vi "DPID.vi"(8 "error in (no error)":errorcluster, 11 "Node Ptr":T2 format="%.0x") -> (0 "error out":errorcluster)   [LabVIEW 2024, in "Diagnostics Addon System Explorer.lvlib"]
uses:
  Diagnostics Addon System Explorer.lvlib
  <vilib>/NI VeriStand/Custom Device API/Custom Device Item Ref.ctl
  Addon Shared/Types/DPID.Rate.ctl
  Types/FG.Action.ctl
  Addon Shared/SubVIs/Constants.vi
  <vilib>/NI/NI VeriStand Advanced SysDef API/SysDef API/SysDef.Property.Set.vi
  <vilib>/NI/NI VeriStand Advanced SysDef API/_SubVIs/SysDef.Property.Set.U32.vi
  <vilib>/NI VeriStand/Custom Device API/NI VeriStand - Get Item Property.vi
  <vilib>/NI VeriStand/Custom Device API/Get Item Property (U32).vi
  <vilib>/NI/NI VeriStand Advanced SysDef API/_SubVIs/SysDef.Property.Set.U32.Array.vi
  <vilib>/NI VeriStand/Custom Device API/Get Item Property (U32 Array).vi
  <vilib>/NI VeriStand/Custom Device Tools/Custom Device Utility Library/NI VeriStand - Search for Item by GUID.vi
  <vilib>/NI VeriStand/Custom Device API/Custom Device API.lvlib
  <vilib>/NI VeriStand/Custom Device Tools/Custom Device Utility Library/Custom Device Utility Library.lvlib
  Addon Shared/Diagnostics Addon Shared.lvlib
panel:
  in  "Speed":T1
  in  "Description":string
  in  "ID":u8 format="%.0x"
  out "PIDs":i32(listbox)
  in  "SHDocVw.IWebBrowser":refnum<k7>(container)
  in  "Header":cluster{"Section Name":string}={"Section Name"="DPID Settings"}
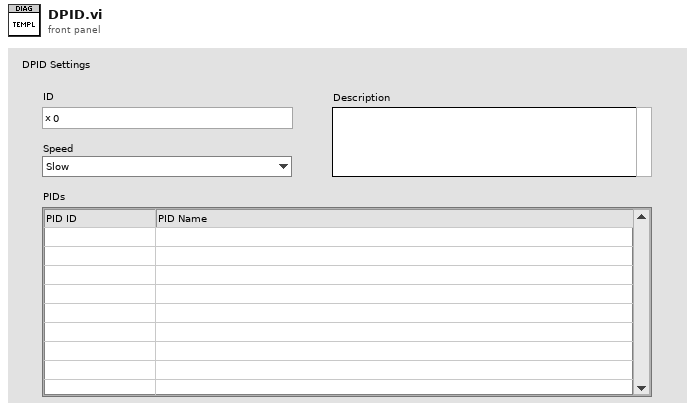
[diagram p1: front panel]
types:
  T1 = typedef "Diagnostics Addon Shared.lvlib/DPID.Rate.ctl" = enum16{"Slow", "Medium", "Fast"}
  T2 = typedef "Custom Device API.lvlib/Custom Device Item Ref.ctl" = u64
  T3 = typedef "Diagnostics Addon System Explorer.lvlib/FG.Action.ctl" = enum16{"Get", "Set"}
  T4 = typedef "Custom Device API.lvlib/Custom Device Item Info.ctl" = cluster{"Name":string, "Is Channel":bool, "GUID":string, "Is Waveform":bool}
  T5 = typedef "Diagnostics Addon Shared.lvlib/DPID.ctl" = cluster{"DPID ID":u8, "Speed":T1, "PIDs":u16[]}
  T6 = typedef "Custom Device API.lvlib/Custom Device Commands.ctl" = enum16{"Default", "Item renamed", "Shutdown", "Dynamic button pressed"}
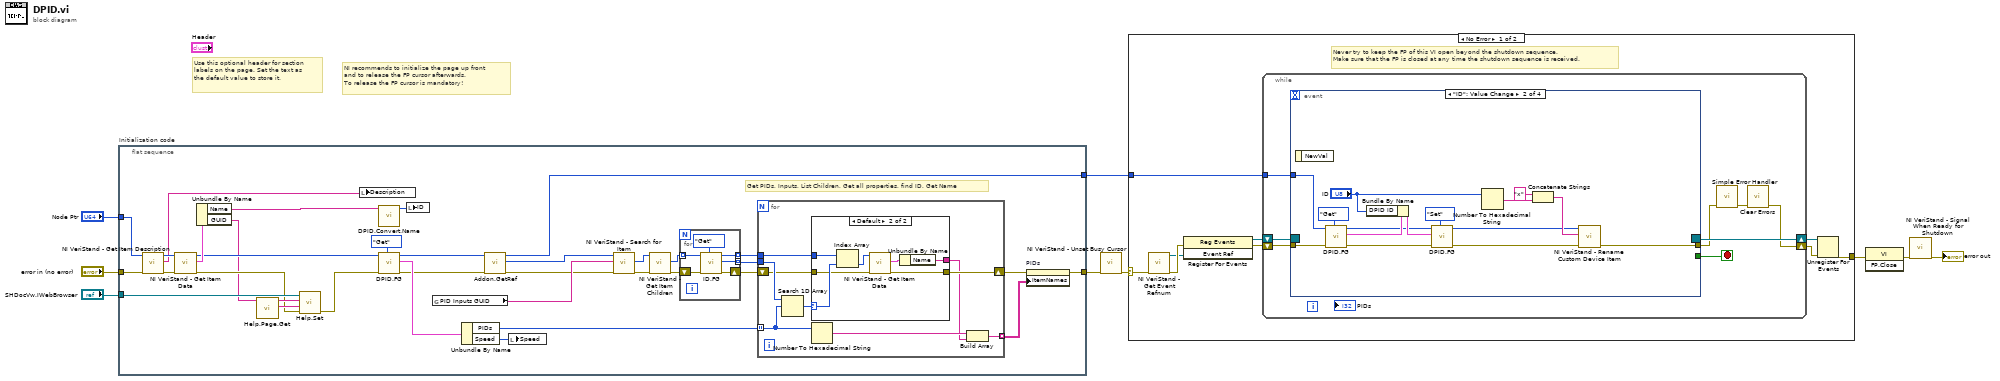
[diagram p0: block diagram]
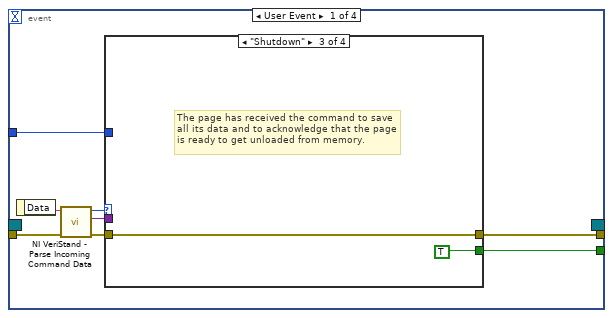
[diagram p2: hidden frame]
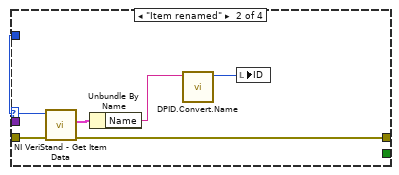
[diagram p4: hidden frame]
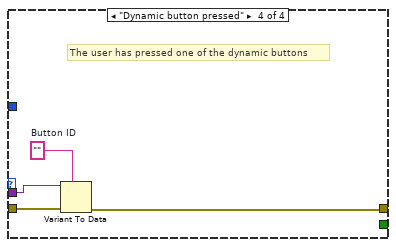
[diagram p5: hidden frame]
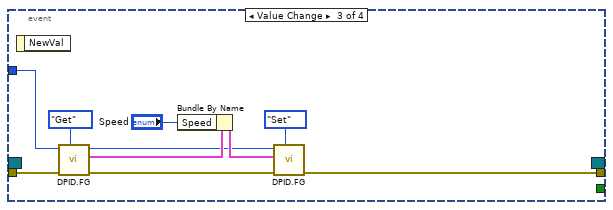
[diagram p6: hidden frame]
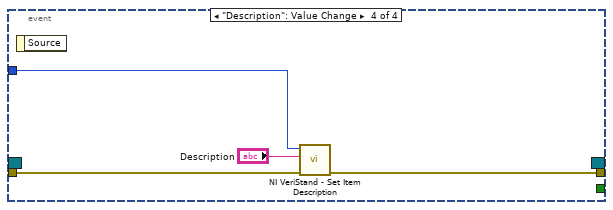
[diagram p7: hidden frame]
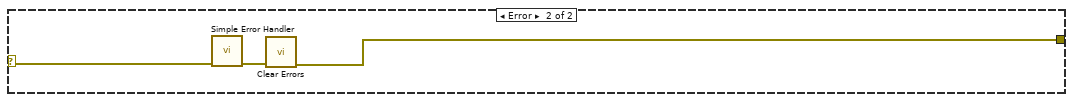
[diagram p8: hidden frame]
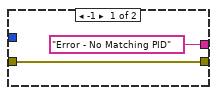
[diagram p9: hidden frame]
diagram:
  # "Use this optional header for section labels on the page. Set the text as the default value to store it."
  # "NI recommends to initialize the page up front\nand to release the FP cursor afterwards.\nTo release the FP cursor is mandatory!"
  n1 = flat-sequence "Initialization code" {
    tunnel: "error in (no error)" -> [w18]
    tunnel: "Node Ptr" -> [w43]
    tunnel: "SHDocVw.IWebBrowser" -> [w39]
    tunnel: [w10] -> w2
    tunnel: [w31] -> w1
    frame #0 {
      # "Get PIDs, Inputs, List Children, Get all properties, find ID, Get Name"
      n2 = call <vilib>:"NI VeriStand - Get Item Description.vi"("error in (no error)"=w18, "Item Ref in"=w43) -> ("error out"=w41:errorcluster, "Description"=w42:string, "Item Ref out"=w44:T2)  [unwired: 7 out]
      n3 = call <vilib>:"NI VeriStand - Get Item Data.vi"("error in (no error)"=w41, "Item Ref in"=w44) -> ("error out"=w17:errorcluster, "Item Info"=w40:T4, "Item Ref out"=w38:T2)  [unwired: 7 out]
      n4 = Unbundle By Name(w40) -> ("Name"=w23:string, "GUID"=w15:string)
      n5 = call "Help.Page.Get.vi"("GUID"=w15) -> ("HTML File"=w20:string, "Main CHM File"=w19:string)  [unwired: 9 in]
      n6 = call "Help.Set.vi"("error in (no error)"=w17, "HTML File"=w20, "Main CHM File"=w19, "SHDocVw.IWebBrowser2"=w39) -> ("error out"=w16:errorcluster)  [unwired: 7 in]
      n7 = local write "Description"(w42) -> ()
      n8 = call "DPID.Convert.Name.vi"("DPID Name"=w23) -> ("DPID ID"=w24:u8)  [unwired: 10 in]
      n9 = call "DPID.FG.vi"("Action"=FG.Action."Get", "error in (no error)"=w16, "Device Item Ref in"=w38) -> ("error out"=w13:errorcluster, "DPID"=w37:T5, "Device Item Ref out"=w14:T2)  [unwired: 6 in]
      n10 = local write "ID"(w24) -> ()
      n11 = global read "Constants.vi" "PID Inputs GUID"() -> (w29:string)
      n12 = Unbundle By Name(w37) -> ("PIDs"=w36:u16[], "Speed"=w22:T1)
      n13 = call "Addon.GetRef.vi"("error in (no error)"=w13, "Node Ptr"=w14) -> ("error out"=w12:errorcluster, "Addon Ref"=w11:T2, "Node Ptr"=w10:T2)  [unwired: 7 in]
      n14 = local write "Speed"(w22) -> ()
      n15 = call-poly <vilib>:"NI VeriStand - Search for Item.vi"("error in"=w12, "Item GUID"=w29, "Section Ref in"=w11) -> ("error out"=w28:errorcluster, "Item Ref"=w26:T2)  [unwired: 5 in, 2 out]
      n16 = call <vilib>:"NI VeriStand - Get Item Children.vi"("error in (no error)"=w28, "Item Ref in"=w26) -> ("error out"=w27:errorcluster, "Child Refs"=w25:T2[])  [unwired: 6 in, 2 out]
      n17 = for {
        tunnel: w25 -> [w68] mode=indexing
        shift-right: [w66] -> w35
        shift-left: w27 -> [w67]
        tunnel: [w65] -> w33 mode=indexing
        tunnel: [w64] -> w34 mode=indexing
        n18 = call "ID.FG.vi"("Action"=FG.Action."Get", "error in (no error)"=w67, "Device Item Ref in"=w68) -> ("error out"=w66:errorcluster, "ID"=w64:u32, "Device Item Ref out"=w65:T2)  [unwired: 6 in]
      }
      n19 = for {
        tunnel: w36 -> [w48] mode=indexing
        shift-right: [w49] -> w32
        shift-left: w35 -> [w50]
        tunnel: w34 -> [w53]
        tunnel: w33 -> [w52]
        tunnel: [w45] -> w30 mode=indexing
        n20 = Search 1D Array(1D array=w53, element=w48) -> (index of element=w51:i32)  [unwired: 1 in]
        n21 = case shown="Default" w51 {
          selector: w51 -> [_ w58]
          tunnel: ["Error - No Matching PID" ("Name") w61] -> w46
          tunnel: [w54 w60] -> w49
          tunnel: w52 -> [_ w59]
          tunnel: w50 -> [w54 w56]
          frame -1 {
          }
          frame Default {
            n22 = Index Array(array=w59, index=w58) -> (element=w57:T2)
            n23 = call <vilib>:"NI VeriStand - Get Item Data.vi"("error in (no error)"=w56, "Item Ref in"=w57) -> ("error out"=w60:errorcluster, "Item Info"=w62:T4)  [unwired: 8 out]
            n24 = Unbundle By Name(w62) -> ("Name"=w61:string)
          }
        }
        n25 = Number To Hexadecimal String(2:w48) -> (0:w47:string)  [unwired: 1 in]
        n26 = Build Array(w47, w46) -> (w45:string[])
      }
      n27 = property on="PIDs" class="MCListbox (strict)"(error in=w32, "ItemNames"=w30) -> (error out=w31:errorcluster)  [unwired: 1 in, 1 out]
    }
  }
  n28 = call <vilib>:"NI VeriStand - Unset Busy Cursor.vi"("error in (no error)"=w1) -> ("error out"=w5:errorcluster)  [unwired: 10 out]
  n29 = case shown="No Error" w5 {
    selector: w5 -> [w69 w138]
    tunnel: [w74 w136] -> w9
    tunnel: w2 -> [w70 _]
    frame No Error {
      # "Never try to keep the FP of this VI open beyond the shutdown sequence.\nMake sure that the FP is closed at any time the shutdown sequence is received."
      n30 = call <vilib>:"NI VeriStand - Get Event Refnum.vi"("error in (no error)"=w69) -> ("error out"=w77:errorcluster, "Event Ref"=w73:refnum<user-event>)  [unwired: 9 out]
      n31 = register-events(error in=w77, w73) -> (reference out=w71:refnum<event-registration>, error out=w72:errorcluster)  [unwired: 1 in]
      n32 = while {
        tunnel: w70 -> [w81]
        shift-right: [w78] -> w75
        shift-left: w72 -> [w84]
        shift-right: [w85] -> w76
        shift-left: w71 -> [w83]
        stop <- w82 stop-if-true
        n33 = event shown="[1] \"ID\": Value Change" {
          selector: w83 -> [_ _ _ _]
          dyn-events: [_ _ _ _] -> w85
          timeout: _ -> [_ _ _ _]
          tunnel: w84 -> [w93 w116 w131 w134]
          tunnel: [w89 _ _ _] -> w82
          tunnel: [w88 w121 w122 w133] -> w80
          tunnel: w81 -> [w87 w114 w130 w135]
          event User Event {
            n34 = event-data() -> ("Data"=w92:string)  [unwired: 1 out]
            n35 = call <vilib>:"NI VeriStand - Parse Incoming Command Data.vi"("error in (no error)"=w93, "Incoming data"=w92) -> ("error out"=w91:errorcluster, "Outgoing data"=w86:variant, "Action"=w90:T6)  [unwired: 7 out]
            n36 = case shown="\"Shutdown\"" w90 {
              tunnel: w91 -> [w94 w100 w101 w106]
              tunnel: [_ _ TRUE _] -> w89
              tunnel: [w94 w97 w101 w103] -> w88
              tunnel: w87 -> [_ w99 _ _]
              tunnel: w86 -> [_ _ _ w105]
              frame "Default", Default {
              }
              frame "Item renamed" {
                n37 = call <vilib>:"NI VeriStand - Get Item Data.vi"("error in (no error)"=w100, "Item Ref in"=w99) -> ("error out"=w97:errorcluster, "Item Info"=w98:T4)  [unwired: 8 out]
                n38 = Unbundle By Name(w98) -> ("Name"=w96:string)
                n39 = call "DPID.Convert.Name.vi"("DPID Name"=w96) -> ("DPID ID"=w95:u8)  [unwired: 10 in]
                n40 = local write "ID"(w95) -> ()
              }
              frame "Shutdown" {
                # "The page has received the command to save all its data and to acknowledge that the page is ready to get unloaded from memory."
              }
              frame "Dynamic button pressed" {
                w104 = ""  # Button ID
                # "The user has pressed one of the dynamic buttons"
                n41 = Variant To Data(error in=w106, type=w104, Variant=w105) -> (error out=w103:errorcluster)  [unwired: 1 out]
              }
            }
          }
          event "ID": Value Change {
            n42 = event-data() -> ()  [unwired: 2 out]
            n43 = call "DPID.FG.vi"("Action"=FG.Action."Get", "error in (no error)"=w116, "Device Item Ref in"=w114) -> ("error out"=w110:errorcluster, "DPID"=w117:T5, "Device Item Ref out"=w108:T2)  [unwired: 6 in]
            n44 = Bundle By Name(cluster=w117, "DPID ID"="ID") -> (w111:T5)
            n45 = call "DPID.FG.vi"("Action"=FG.Action."Set", "error in (no error)"=w110, "DPID"=w111, "Device Item Ref in"=w108) -> ("error out"=w109:errorcluster, "Device Item Ref out"=w107:T2)  [unwired: 5 in, 1 out]
            n46 = Number To Hexadecimal String(2:"ID") -> (0:w120:string)  [unwired: 1 in]
            n47 = Concatenate Strings("x" ("element"), w120) -> (w118:string)
            n48 = call <vilib>:"NI VeriStand - Rename Custom Device Item.vi"("error in (no error)"=w109, "New Name"=w118, "Item Ref in"=w107) -> ("error out"=w121:errorcluster)  [unwired: 1 in, 7 out]
          }
          event Value Change {
            n49 = event-data() -> ()  [unwired: 2 out]
            n50 = call "DPID.FG.vi"("Action"=FG.Action."Get", "error in (no error)"=w131, "Device Item Ref in"=w130) -> ("error out"=w123:errorcluster, "DPID"=w129:T5, "Device Item Ref out"=w124:T2)  [unwired: 6 in]
            n51 = Bundle By Name(cluster=w129, "Speed"="Speed") -> (w125:T5)
            n52 = call "DPID.FG.vi"("Action"=FG.Action."Set", "error in (no error)"=w123, "DPID"=w125, "Device Item Ref in"=w124) -> ("error out"=w122:errorcluster)  [unwired: 5 in, 2 out]
          }
          event "Description": Value Change {
            n53 = event-data() -> ()  [unwired: 2 out]
            n54 = call <vilib>:"NI VeriStand - Set Item Description.vi"("error in (no error)"=w134, "Description"="Description", "Item Ref in"=w135) -> ("error out"=w133:errorcluster)  [unwired: 8 out]
          }
        }
        n55 = call <vilib>:"Simple Error Handler.vi"("error in (no error)"=w80) -> ("error out"=w79:errorcluster)  [unwired: 1 in, 7 out]
        n56 = call <vilib>:"Clear Errors.vi"("error in (no error)"=w79) -> ("error out"=w78:errorcluster)  [unwired: 1 in, 5 out]
      }
      n57 = Unregister For Events(event registration refnum=w76, error in=w75) -> (error out=w74:errorcluster)
    }
    frame Error {
      n58 = call <vilib>:"Simple Error Handler.vi"("error in (no error)"=w138) -> ("error out"=w137:errorcluster)  [unwired: 1 in, 7 out]
      n59 = call <vilib>:"Clear Errors.vi"("error in (no error)"=w137) -> ("error out"=w136:errorcluster)  [unwired: 1 in, 5 out]
    }
  }
  n60 = invoke class="VI" method="FP.Close"(error in=w9) -> (error out=w8:errorcluster)  [unwired: 2 in, 2 out]
  n61 = call <vilib>:"NI VeriStand - Signal When Ready for Shutdown.vi"("error in (no error)"=w8) -> ("error out"=→"error out":errorcluster)  [unwired: 10 out]
